vi "Fill DataSet.vi"(8 "error in (no error)":errorcluster caption="错误输入（无错误）", 10 "srcTable":string, 11 "OleDBClass 输入":refnum<class "OleDBClass.lvclass"> caption="DNL_LabVIEW Object in") -> (0 "error out":errorcluster caption="错误输出", 3 "OleDBClass 输出":refnum<class "OleDBClass.lvclass"> caption="DNL_LabVIEW Object out")   [LabVIEW 2012, in "OleDBClass.lvclass"]
uses:
  OleDBClass.lvclass
  OleDBClass.lvclass/OleDBClass.ctl
  System.Data
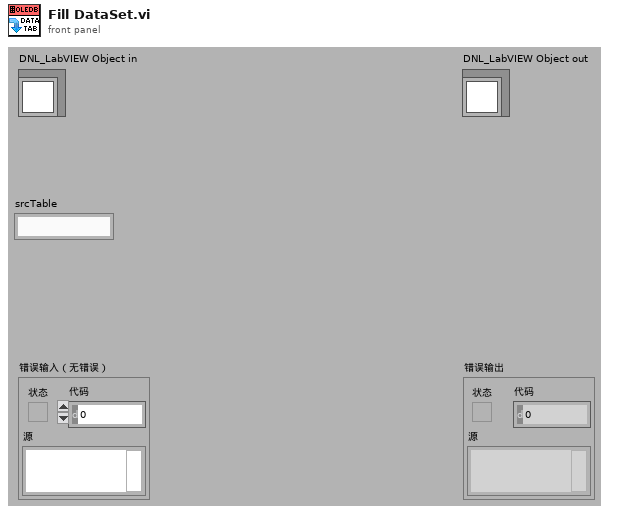
[diagram p1: front panel]
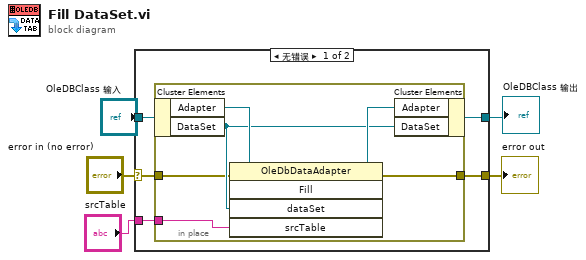
[diagram p0: block diagram]
diagram:
  n1 = case shown="无错误" "error in (no error)" {
    selector: "error in (no error)" -> [w8 w18]
    tunnel: [w7 w18] -> w4
    tunnel: [w9 w17] -> w2
    tunnel: "OleDBClass 输入" -> [w10 w17]
    tunnel: "srcTable" -> [w6 _]
    frame No Error {
      n2 = in-place {
        in-place-border: w8 -> [w13]
        in-place-border: [w12] -> w7
        in-place-border: w6 -> [w11]
        n3 = in-place-cluster #1(w10) -> ("Adapter"=w16:refnum<k24>, "DataSet"=w14:refnum<k24>)
        n4 = invoke class="OleDbDataAdapter" method="Fill"(reference=w16, error in=w13, "dataSet"=w14, "srcTable"=w11) -> (reference out=w15:refnum<k24>, error out=w12:errorcluster)  [unwired: 1 in, 3 out]
        n5 = in-place-cluster #1("Adapter"=w15, "DataSet"=w14) -> (w9:refnum<class "OleDBClass.lvclass">)
      }
    }
    frame Error {
    }
  }
  "error out" <- w4
  "OleDBClass 输出" <- w2
